vi "Pre Launch Init.vi"(11 "ExampleSimpleRootModel in":refnum<class "SimpleRootModel.lvclass">) -> (0 "error out":errorcluster, 3 "ExampleSimpleRootModel out":refnum<class "SimpleRootModel.lvclass">)   [LabVIEW 2017, in "MVAExamples.lvlib" / "SimpleRootModel.lvclass"]
doc: "(<B>Filename</B>: Actor Framework.lvlib:Actor.lvclass:Pre Launch Init.vi)\n\nDefines behavior that occurs after the Launch Nested Actor method is invoked but before the actor's Actor Core method begins running.\n\nBy default, this method does nothing. A descendant class may override it to define behavior."
uses:
  SimpleRootModel.lvclass
  C:/Git/mva-framework/Source/Framework/IObserver/IObserver/IObserver.lvclass
  C:/Program Files (x86)/National Instruments/LabVIEW 2017/vi.lib/ActorFramework/Actor/Actor.lvclass
  SimpleRootModel.lvclass/SimpleRootModel.ctl
  <vilib>/ActorFramework/Actor/Actor.lvclass/Actor.ctl
  <vilib>/ActorFramework/Message Enqueuer/Message Enqueuer.lvclass/Message Enqueuer.ctl
  ExampleSimpleRootModel Messages/Execute State Msg/Execute State Msg.lvclass/Execute State Msg.ctl
  <vilib>/ActorFramework/Message Enqueuer/Init from Existing Queue.vi
  <vilib>/ActorFramework/Message Enqueuer/Enqueue.vi
  ExampleSimpleRootModel Messages/Execute State Msg/Execute State Msg.lvclass
  C:/Program Files (x86)/National Instruments/LabVIEW 2017/vi.lib/ActorFramework/Message/Message.lvclass
  <vilib>/ActorFramework/Message Priority Queue/Priority Enqueue.vi
  Source/Framework/IModel/IModel/IModel.lvclass
  <vilib>/ActorFramework/Message Enqueuer/Message Enqueuer.lvclass
  Source/Framework/IObserver/IObserver/IObserver.lvclass
  <vilib>/ActorFramework/Actor/Actor.lvclass
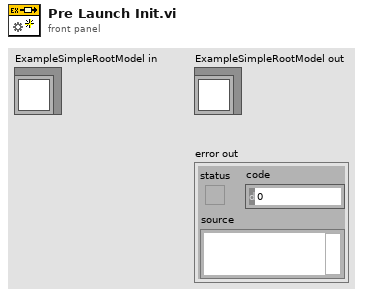
[diagram p1: front panel]
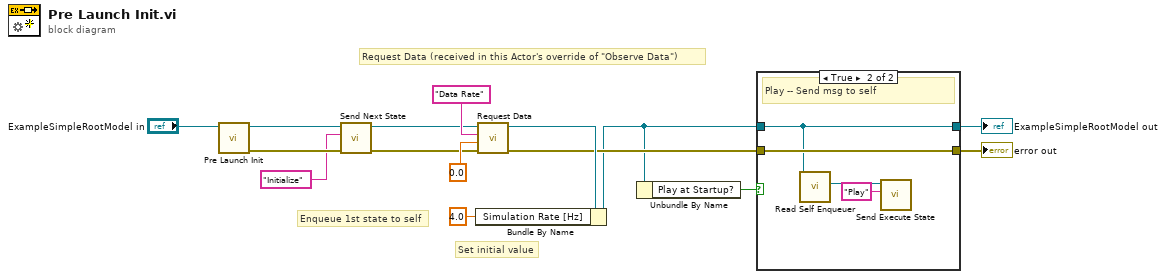
[diagram p0: block diagram]
diagram:
  # "Request Data (received in this Actor's override of \"Observe Data\")"
  # "Set initial value"
  # "Enqueue 1st state to self"
  n1 = call-parent "Pre Launch Init.vi"("IModel in"="ExampleSimpleRootModel in") -> ("error out"=w15:errorcluster, "IModel out"=w13:refnum<class "SimpleRootModel.lvclass">)  [unwired: 9 in]
  n2 = call "Send Next State.vi"("error in (no error)"=w15, "State"="Initialize", "ExampleSimpleRootModel in"=w13) -> ("error out"=w6:errorcluster, "ExampleSimpleRootModel out"=w7:refnum<class "SimpleRootModel.lvclass">)  [unwired: 7 in]
  n3 = call "Request Data.vi"("error in (no error)"=w6, "Data Type"=0.0, "Datum Name"="Data Rate", "IObserver in"=w7) -> ("error out"=w4:errorcluster, "IObserver out"=w11:refnum<class "SimpleRootModel.lvclass">)  [unwired: 5 in, 1 out]
  n4 = Bundle By Name(cluster=w11, "Simulation Rate [Hz]"=4.0) -> (w3:refnum<class "SimpleRootModel.lvclass">)
  n5 = Unbundle By Name(w3) -> ("Play at Startup?"=w5:bool)
  n6 = case shown="True" w5 {
    tunnel: w4 -> [w16 w21]
    tunnel: w3 -> [w17 w20]
    tunnel: [w17 w20] -> w2
    tunnel: [w16 w21] -> w1
    frame False {
      # "Wait for external msg"
      # "Do nothing"
    }
    frame True {
      # "Play -- Send msg to self"
      n7 = call <vilib>:"Read Self Enqueuer.vi"("Actor"=w20) -> ("Self Enqueuer"=w19:refnum<class "Message Enqueuer.lvclass">)  [unwired: 10 in]
      n8 = call "Send Execute State.vi"("State"="Play", "Message Enqueuer"=w19) -> ()  [unwired: 8 in, 2 out]
    }
  }
  "error out" <- w1
  "ExampleSimpleRootModel out" <- w2
